vi "Update Target Angle.vi"(8 "Turret Position":dbl, 9 "Deadband":dbl, 10 "Tx":dbl) -> ()   [LabVIEW 2019]
uses:
  <vilib>/Rock Robotics/Network Tables/NT Read Number.vi
  Framework/Robot Global Data.vi
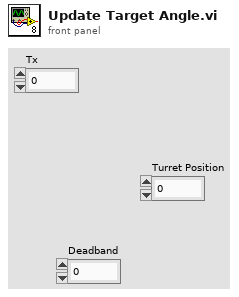
[diagram p1: front panel]
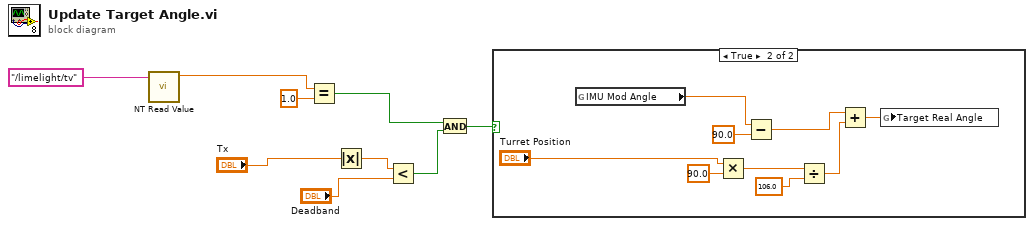
[diagram p0: block diagram]
diagram:
  n1 = call-poly <vilib>:"NT Read Value.vi"("Name"="/limelight/tv") -> ("Numeric"=w8:dbl)  [unwired: 9 in, 1 out]
  n2 = Equal?(x=w8, y=1.0) -> (x = y?=w6:bool)
  n3 = Absolute Value(x="Tx") -> (abs(x)=w4:dbl)
  n4 = Less?(x=w4, y="Deadband") -> (x < y?=w2:bool)
  n5 = And(x=w6, y=w2) -> (x .and. y?=w1:bool)
  n6 = case shown="True" w1 {
    frame False {
    }
    frame True {
      n7 = global read "Robot Global Data.vi" "IMU Mod Angle"() -> (w12:dbl)
      n8 = Multiply(x="Turret Position", y=90.0) -> (x*y=w18:dbl)
      n9 = Subtract(x=w12, y=90.0) -> (x-y=w10:dbl)
      n10 = Divide(x=w18, y=106.0) -> (x/y=w14:dbl)
      n11 = Add(x=w10, y=w14) -> (x+y=w13:dbl)
      n12 = global write "Robot Global Data.vi" "Target Real Angle"(w13) -> ()
    }
  }
